vi "2810A Parse Scan List.vi"(10 "ApplicationNumberOfWeldChannels":i32, 11 "Matrix Input String":string="ch0:6") -> (3 "Channel Array":string[](array[string]))   [LabVIEW 2019, in "SupportVIs.lvlib"]
uses:
  SupportVIs.lvlib
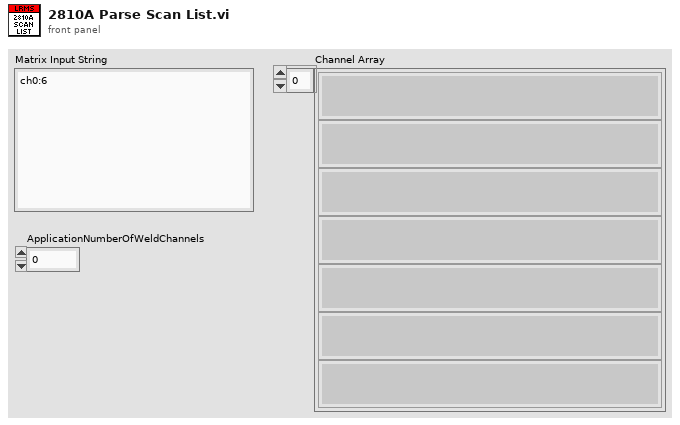
[diagram p1: front panel]
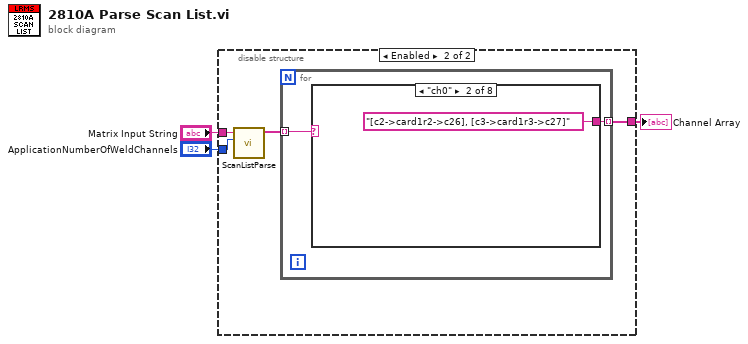
[diagram p0: block diagram]
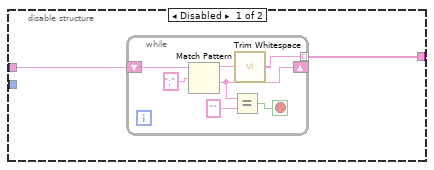
[diagram p2: hidden frame]
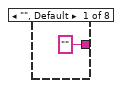
[diagram p3: hidden frame]
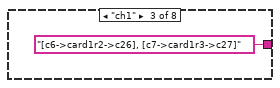
[diagram p4: hidden frame]
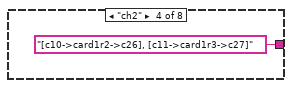
[diagram p5: hidden frame]
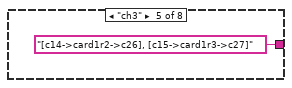
[diagram p6: hidden frame]
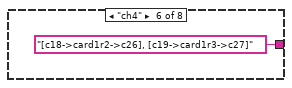
[diagram p7: hidden frame]
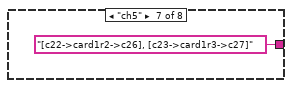
[diagram p8: hidden frame]
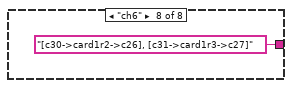
[diagram p9: hidden frame]
diagram:
  n1 = disable-structure shown="Enabled" {
    disable-tunnel: "Matrix Input String" -> [w5 w15]
    disable-tunnel: [w4 w14] -> w2
    disable-tunnel: "ApplicationNumberOfWeldChannels" -> [_ w13]
    frame Disabled {
      n2 = while {
        tunnel: [w6] -> w4 mode=indexing
        shift-right: [w8] -> _
        shift-left: w5 -> [w11]
        stop <- w10 stop-if-true
        n3 = Match Pattern(string=w11, regular expression=";" ("search string")) -> (before substring=w7:string, after substring=w8:string)  [unwired: 1 in, 2 out]
        n4 = Equal?(x=w8, y="") -> (x = y?=w10:bool)
        n5 = call <vilib>:"Trim Whitespace.vi"("string"=w7) -> ("trimmed string"=w6:string)  [unwired: 1 in]
      }
    }
    frame Enabled {
      n6 = call "ScanListParse.vi"("ApplicationNumberOfWeldChannels"=w13, "Input"=w15) -> ("Output"=w16:string[])  [unwired: 9 in]
      n7 = for {
        tunnel: w16 -> [w18] mode=indexing
        tunnel: [w17] -> w14 mode=indexing
        n8 = case shown="\"ch0\"" w18 {
          tunnel: ["" "[c2->card1r2->c26], [c3->card1r3->c27]" "[c6->card1r2->c26], [c7->card1r3->c27]" "[c10->card1r2->c26], [c11->card1r3->c27]" "[c14->card1r2->c26], [c15->card1r3->c27]" "[c18->card1r2->c26], [c19->card1r3->c27]" "[c22->card1r2->c26], [c23->card1r3->c27]" "[c30->card1r2->c26], [c31->card1r3->c27]"] -> w17
          frame "", Default {
          }
          frame "ch0" {
          }
          frame "ch1" {
          }
          frame "ch2" {
          }
          frame "ch3" {
          }
          frame "ch4" {
          }
          frame "ch5" {
          }
          frame "ch6" {
          }
        }
      }
    }
  }
  "Channel Array" <- w2
